vi "setStrain.vi"(6 "Channel":i32=1 min=1 max=2, 8 "error in (no error)":errorcluster, 9 "Slew (V/s)":dbl, 10 "Strain (V)":dbl, 11 "Inst.RP100 in":refnum<class "Inst.RP100.lvclass">) -> (0 "error out":errorcluster, 3 "Inst.RP100 out":refnum<class "Inst.RP100.lvclass">)   [LabVIEW 2019, in "Inst.RP100.lvlib" / "Inst.RP100.lvclass"]
doc: "Set the output <b>Strain</b> with <b>Slew</b> such that Channel 1 = -Channel 2. \n\n<b>Output Channel</b> is not used."
uses:
  Inst.RP100.lvclass
  <userlib>/LevyLab/Instrument Framework/Instrument Types/Strain/Instrument.Strain.lvclass
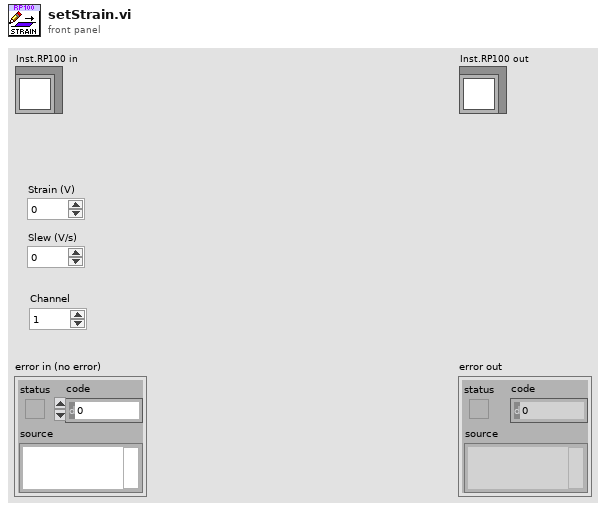
[diagram p1: front panel]
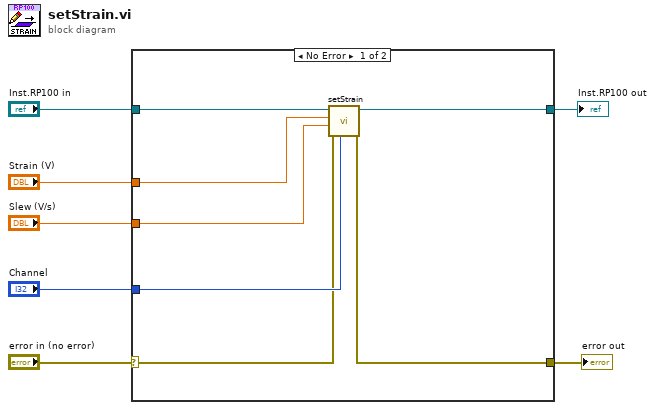
[diagram p0: block diagram]
diagram:
  n1 = case shown="No Error" "error in (no error)" {
    selector: "error in (no error)" -> [w8 w16]
    tunnel: [w10 w16] -> w6
    tunnel: "Strain (V)" -> [w13 _]
    tunnel: "Inst.RP100 in" -> [w14 w15]
    tunnel: [w11 w15] -> w3
    tunnel: "Slew (V/s)" -> [w12 _]
    tunnel: "Channel" -> [w9 _]
    frame No Error {
      n2 = call-parent "setStrain.vi"("Channel"=w9, "error in (no error)"=w8, "Slew (V/s)"=w12, "Strain (V)"=w13, "Instrument.Strain in"=w14) -> ("error out"=w10:errorcluster, "Instrument.Strain out"=w11:refnum<class "Inst.RP100.lvclass">)  [unwired: 5 in]
    }
    frame Error {
    }
  }
  "error out" <- w6
  "Inst.RP100 out" <- w3
